vi "two action.vi"() -> ()   [LabVIEW 2017]
uses:
  tools/queue/subvi/initMultiple.vi
  tools/queue/subvi/sendMultiple.vi
  tools/queue/subvi/sendSingle.vi
  tools/queue/subvi/readMultiple.vi
  tools/queue/subvi/dataUnpackBool.vi
panel:
  in  "停止":bool
  in  "B":bool
  in  "A":bool
  out "B_action":string
  out "A_action":string
  out "B_action":bool=TRUE
  out "A_action":bool=TRUE
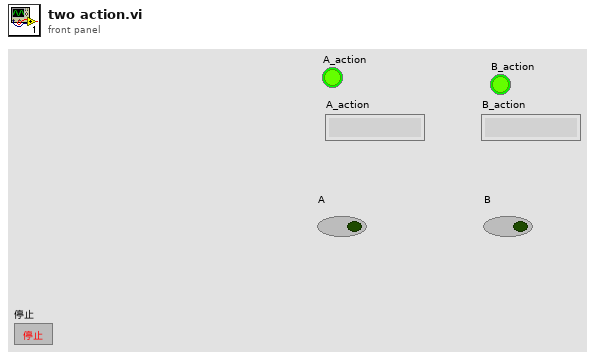
[diagram p1: front panel]
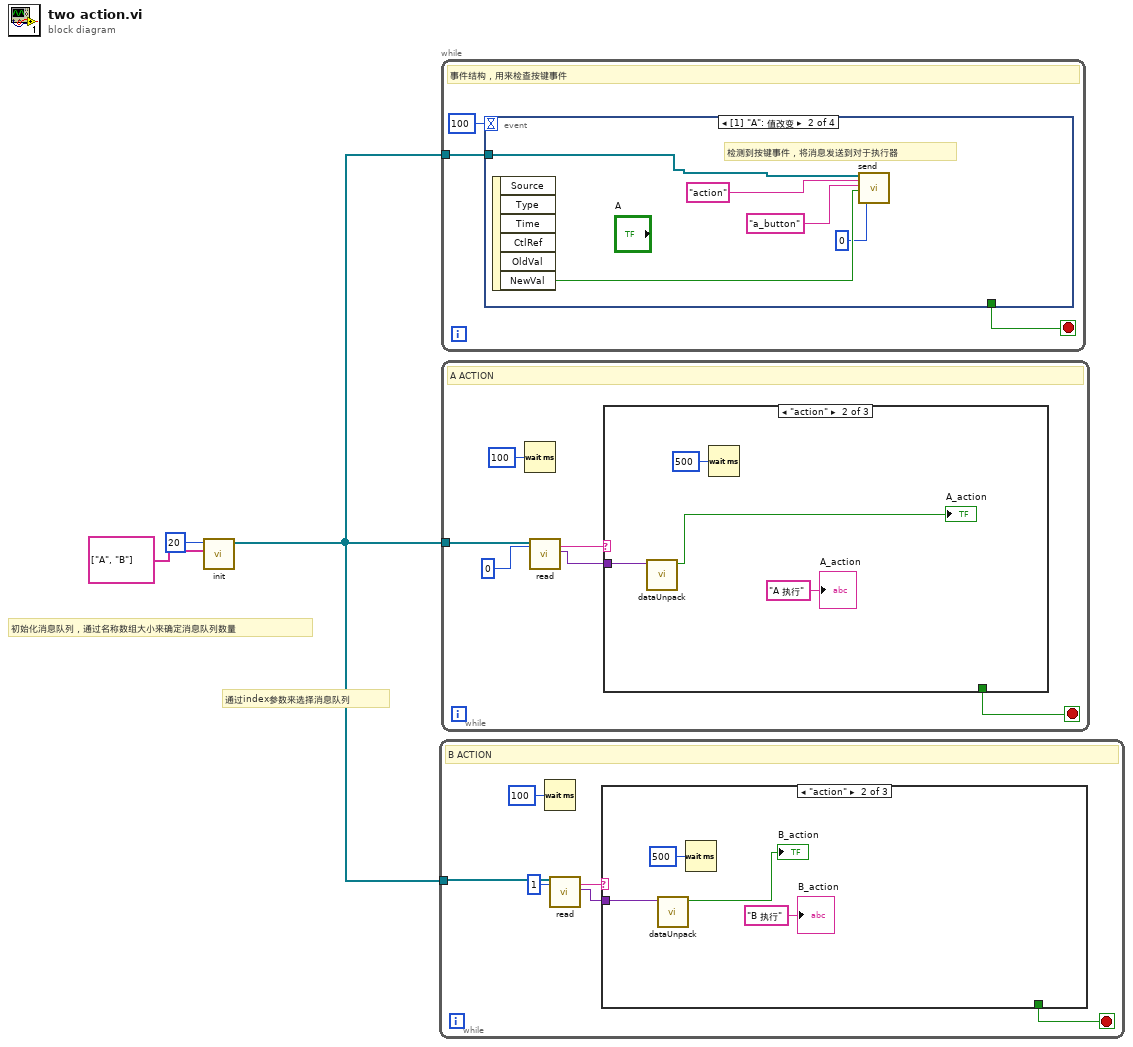
[diagram p0: block diagram]
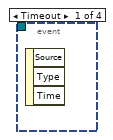
[diagram p2: hidden frame]
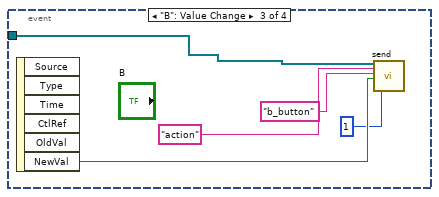
[diagram p3: hidden frame]
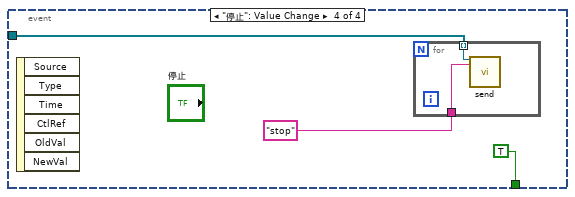
[diagram p4: hidden frame]
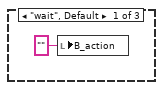
[diagram p5: hidden frame]
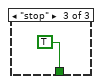
[diagram p6: hidden frame]
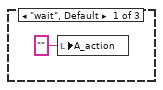
[diagram p7: hidden frame]
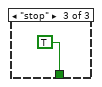
[diagram p8: hidden frame]
diagram:
  # "通过index参数来选择消息队列"
  # "初始化消息队列，通过名称数组大小来确定消息队列数量"
  n1 = call-poly "init.vi"("name"=string[] ["A", "B"], "size(-1)"=20) -> ("refer"=w1:refnum<queue>[])  [unwired: 8 in, 1 out]
  n2 = while {
    tunnel: w1 -> [w5]
    stop <- w7 stop-if-true
    # "B ACTION"
    n3 = Wait (ms)(milliseconds to wait=u32 100 ("等待时间（毫秒）")) -> ()  [unwired: 1 out]
    n4 = call-poly "read.vi"("refer"=w5, "Index"=1) -> ("to"=w8:string, "data"=w6:variant)  [unwired: 10 in, 6 out]
    n5 = case shown="\"action\"" w8 {
      tunnel: [_ _ TRUE] -> w7
      tunnel: w6 -> [_ w12 _]
      frame "wait", Default {
        n6 = local write "B_action"("" ("B_action")) -> ()
      }
      frame "action" {
        n7 = call-poly "dataUnpack.vi"("data"=w12) -> ("bool"=→"B_action":bool)  [unwired: 9 in, 1 out]
        n8 = Wait (ms)(milliseconds to wait=u32 500 ("等待时间（毫秒）")) -> ()  [unwired: 1 out]
        "B_action" <- "B 执行" ("B_action")
      }
      frame "stop" {
      }
    }
  }
  n9 = while {
    tunnel: w1 -> [w17]
    stop <- w16 stop-if-true
    # "事件结构，用来检查按键事件"
    n10 = event shown="[1] \"A\": 值改变" {
      selector: _ -> [_ _ _ _]
      dyn-events: _ -> [_ _ _ _]
      timeout: 100 -> [_ _ _ _]
      tunnel: w17 -> [_ w20 w25 w29]
      tunnel: [_ _ _ TRUE] -> w16
      event Timeout {
        n11 = event-data() -> ()  [unwired: 1 in, 3 out]
      }
      event "A": Value Change {
        # "检测到按键事件，将消息发送到对于执行器"
        n12 = event-data() -> ("NewVal"=w21:bool)  [unwired: 1 in, 5 out]
        n13 = call-poly "send.vi"("refer"=w20, "to"="action", "from"="a_button", "data"=w21, "Index"=0) -> ()  [unwired: 13 in, 2 out]
      }
      event "B": Value Change {
        n14 = event-data() -> ("NewVal"=w26:bool)  [unwired: 1 in, 5 out]
        n15 = call-poly "send.vi"("refer"=w25, "to"="action" ("to 2"), "from"="b_button", "data"=w26, "Index"=1) -> ()  [unwired: 13 in, 2 out]
      }
      event "停止": Value Change {
        n16 = event-data() -> ()  [unwired: 1 in, 6 out]
        n17 = for {
          tunnel: "stop" ("to 2") -> [w33]
          tunnel: w29 -> [w32] mode=indexing
          n18 = call-poly "send.vi"("refer"=w32, "to"=w33) -> ()  [unwired: 16 in, 2 out]
        }
      }
    }
  }
  n19 = while {
    tunnel: w1 -> [w35]
    stop <- w37 stop-if-true
    # "A ACTION"
    n20 = Wait (ms)(milliseconds to wait=u32 100 ("等待时间（毫秒）")) -> ()  [unwired: 1 out]
    n21 = call-poly "read.vi"("refer"=w35, "Index"=0) -> ("to"=w38:string, "data"=w36:variant)  [unwired: 10 in, 6 out]
    n22 = case shown="\"action\"" w38 {
      tunnel: [_ _ TRUE] -> w37
      tunnel: w36 -> [_ w42 _]
      frame "wait", Default {
        n23 = local write "A_action"("" ("A_action")) -> ()
      }
      frame "action" {
        n24 = call-poly "dataUnpack.vi"("data"=w42) -> ("bool"=→"A_action":bool)  [unwired: 9 in, 1 out]
        n25 = Wait (ms)(milliseconds to wait=u32 500 ("等待时间（毫秒）")) -> ()  [unwired: 1 out]
        "A_action" <- "A 执行" ("A_action")
      }
      frame "stop" {
      }
    }
  }
